vi "Request-Reply_TEMPLATE.vi"(8 "error in (no error)":errorcluster, 10 "Parameters":variant, 11 "SMO.jsonRPC":refnum<class "SMO.jsonRPC.lvclass">) -> (0 "error out":errorcluster, 1 "id":i32, 3 "SMO.jsonRPC out":refnum<class "SMO.jsonRPC.lvclass">)   [LabVIEW 2013, in "SMO.jsonRPC.lvclass"]
doc: "---------------------------------------------------------------\nJKI State Machine Objects™\nhttp://jki.net/state-machine-objects/\nCopyright (C) 2005-2015, JKI <info@jki.net>\nALL RIGHTS RESERVEDJKI State Machine Objects (SMO) 1.0.0.5\nJKI - JKI\nCopyright (c) 2016, JKI"
uses:
  SMO.jsonRPC.lvclass
panel:
  # "For instructions on how to use the JKI State Machine Objects, examples and video tutorials, visit:\nhttp://jki.net/state-machine-objects/\n\nJKI State Machine Objects™\nhttp://jki.net/state-machine-objects/\nCopyright (C) 2005-2015, JKI <info@jki.net>\nALL RIGHTS RESERVED"
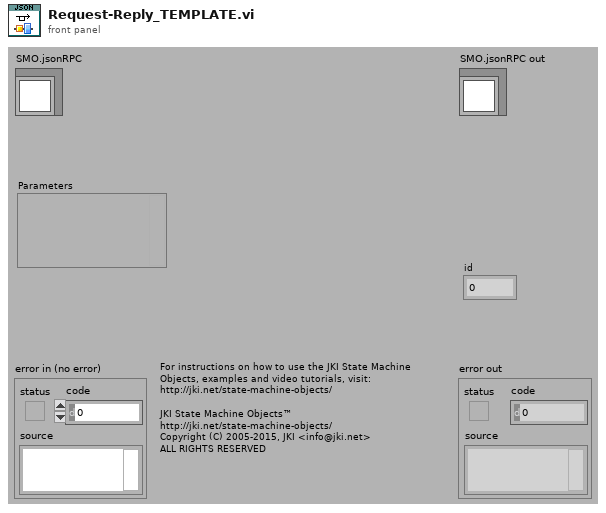
[diagram p1: front panel]
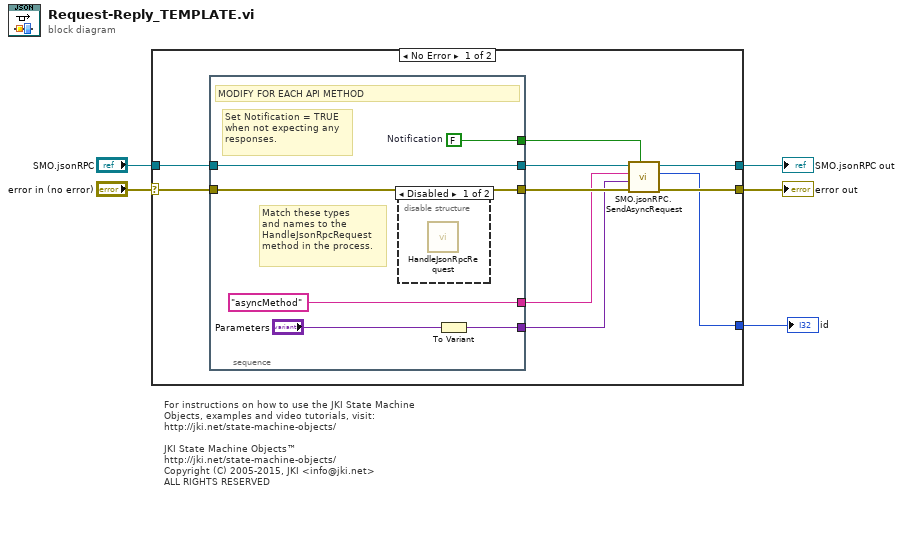
[diagram p0: block diagram]
diagram:
  # "For instructions on how to use the JKI State Machine Objects, examples and video tutorials, visit:\nhttp://jki.net/state-machine-objects/\n\nJKI State Machine Objects™\nhttp://jki.net/state-machine-objects/\nCopyright (C) 2005-2015, JKI <info@jki.net>\nALL RIGHTS RESERVED"
  n1 = case shown="No Error" "error in (no error)" {
    selector: "error in (no error)" -> [w10 w22]
    tunnel: "SMO.jsonRPC" -> [w11 w23]
    tunnel: [w14 w22] -> w4
    tunnel: [w15 w23] -> w3
    tunnel: [w13 _] -> w1
    frame No Error {
      n2 = stacked-sequence {
        tunnel: ["asyncMethod" ("Method")] -> w7
        tunnel: [w19] -> w6
        tunnel: [w20] -> w12
        tunnel: w11 -> [w20]
        tunnel: [w18] -> w8
        tunnel: w10 -> [w16]
        tunnel: [w16] -> w9
        frame #0 {
          w18 = FALSE  # Notification
          # "Set Notification = TRUE\nwhen not expecting any\nresponses."
          # "Match these types\nand names to the\nHandleJsonRpcRequest\nmethod in the process."
          # "MODIFY FOR EACH API METHOD"
          n3 = disable-structure shown="Disabled" {
            frame Disabled {
              n4 = call "HandleJsonRpcRequest.vi"() -> ()  [unwired: 9 in, 3 out]
            }
            frame Enabled {
            }
          }
          n5 = To Variant(anything="Parameters") -> (Variant=w19:variant)
        }
      }
      n6 = call "SMO.jsonRPC.SendAsyncRequest.vi"("Notification"=w8, "error in (no error)"=w9, "Parameters"=w6, "Method"=w7, "SMO.jsonRPC in"=w12) -> ("error out"=w14:errorcluster, "id"=w13:i32, "SMO.jsonRPC out"=w15:refnum<class "SMO.jsonRPC.lvclass">)  [unwired: 4 in]
    }
    frame Error {
    }
  }
  "error out" <- w4
  "SMO.jsonRPC out" <- w3
  "id" <- w1
